vi "Listbox.Init.vi"(8 "error in (no error)":errorcluster, 9 "Config":T1, 10 "Caption.Text":string, 11 "Listbox":refnum<vi>) -> (0 "error out":errorcluster, 3 "Listbox":refnum<vi>)   [LabVIEW 2015, in "Workspace.Obejct.Radio.lvlib"]
uses:
  Workspace.Obejct.Radio.lvlib
  Types/Config.ctl
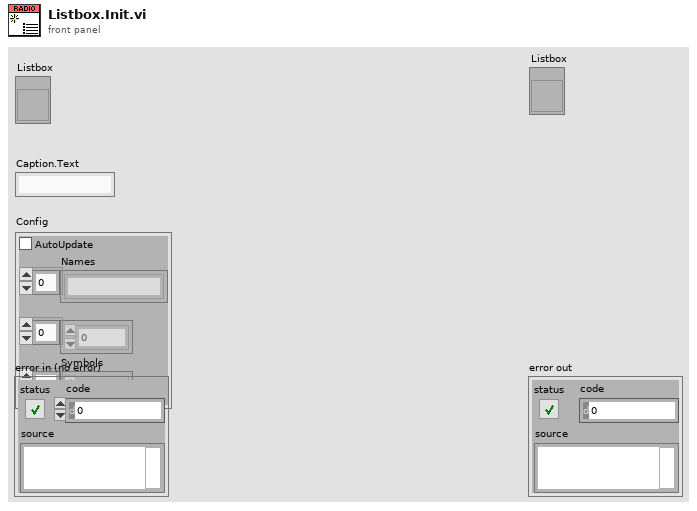
[diagram p1: front panel]
types:
  T1 = typedef "Workspace.Obejct.Radio.lvlib/Config.ctl" = cluster{"AutoUpdate":bool, "Names":string[], "Values":dbl[], "Symbols":i32[]}
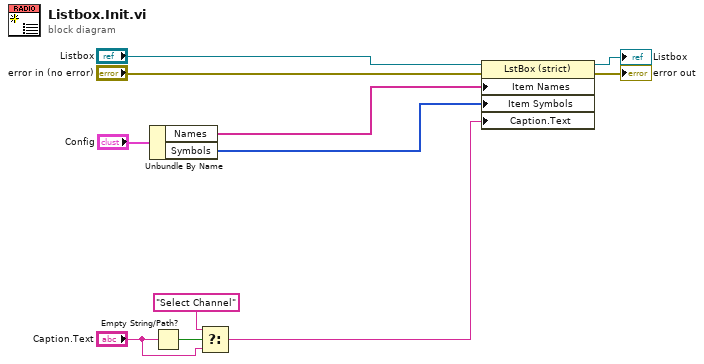
[diagram p0: block diagram]
diagram:
  n1 = Unbundle By Name("Config") -> ("Names"=w2:string[], "Symbols"=w1:i32[])
  n2 = Empty String/Path?(string/path="Caption.Text") -> (empty?=w6:bool)
  n3 = Select(t="Select Channel", s=w6, f="Caption.Text") -> (s? t:f=w3:string)
  n4 = property class="LstBox (strict)"(reference="Listbox", error in="error in (no error)", "Item Names"=w2, "Item Symbols"=w1, "Caption.Text"=w3) -> (reference out=→"Listbox":refnum<vi>, error out=→"error out":errorcluster)
